vi "TestToff.vi"() -> ()   [LabVIEW 2022 SP3]
panel:
  out "elapsed time (ms)":i32
  in  "Ton":i32=1000
  in  "input":bool
  out "Waveform Chart":u8(graph)
  in  "stop":bool
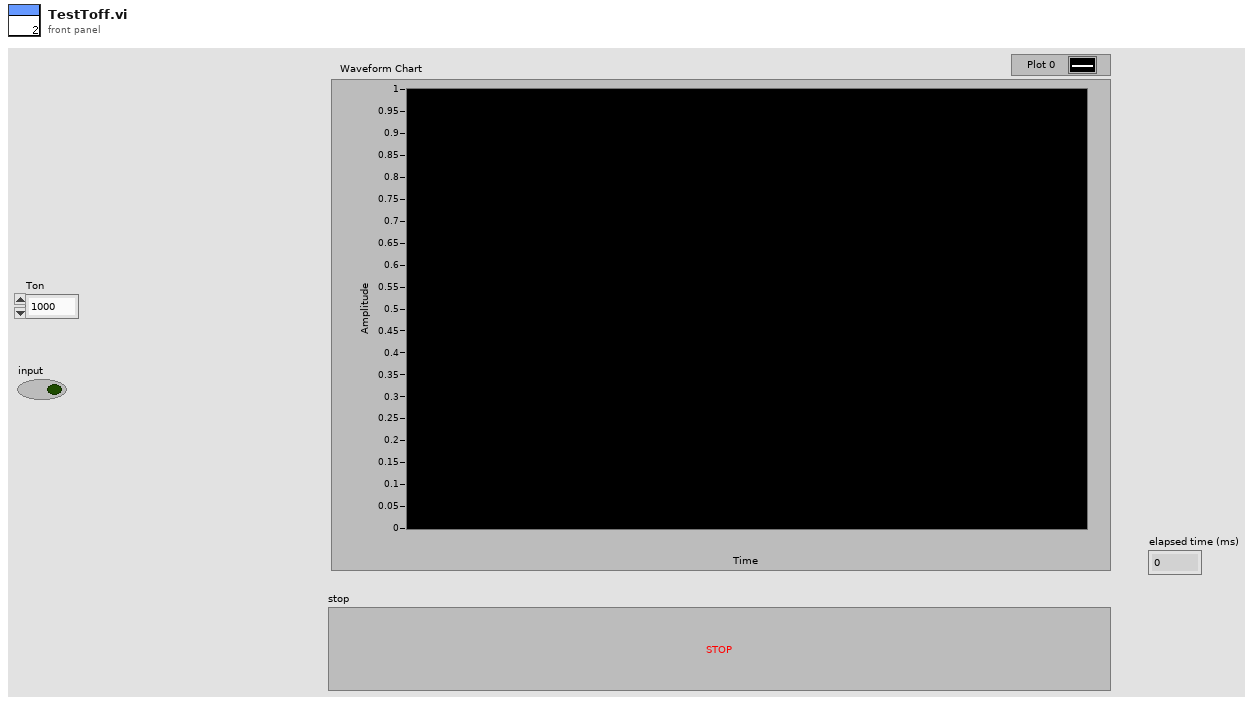
[diagram p1: front panel]
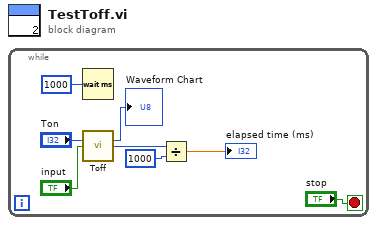
[diagram p0: block diagram]
diagram:
  n1 = while {
    stop <- "stop" stop-if-true
    n2 = Wait (ms)(milliseconds to wait=u32 1000) -> ()  [unwired: 1 out]
    n3 = call "Toff.vi"("preset time (ms)"="Ton", "input"="input") -> ("off"=→"Waveform Chart":u8, "elapsed time (ms)"=w3:i32)  [unwired: 11 in, 1 out]
    n4 = Divide(x=w3, y=1000) -> (x/y=→"elapsed time (ms)":dbl)
  }
